vi "7-19-19 increasing temp.vi"() -> ()   [LabVIEW 2016]
uses:
  <userlib>/Levylab/LV to ITX/LVtoITX.lvclass
  <vilib>/Analysis/NI_AALPro.lvlib
panel:
  out "G Vs Time 2":cluster{"Data":dbl[], "Data":dbl[]}(graph)
  in  "Path 2":path=path "G:/My Drive/Data/SA40060.20190715.000000.dat"
  out "dG/dt Vs Temp Normalized vs prev":cluster{"Data":dbl[], "Data":dbl[]}[](graph)
  out "dG/dt Vs Temp Normalized vs 275K":cluster{"Data":dbl[], "Data":dbl[]}[](graph)
  out "dG/dt Vs Temp":cluster{"Data":dbl[], "Data":dbl[]}[](graph)
  out "output cluster":cluster{dbl[], dbl[], dbl[], dbl[]}
  out "G2T Vs Temp":cluster{"Data":dbl[], "Data":dbl[]}[](graph)
  out "Data":dbl[][](array[numeric])
  out "G Vs Time":cluster{"Data":dbl[], "Data":dbl[]}[](graph)
  out "Wavenames":string[](array[string])
  in  "Path":path=path "G:/My Drive/Data/SA40060.20190715.000000.dat"
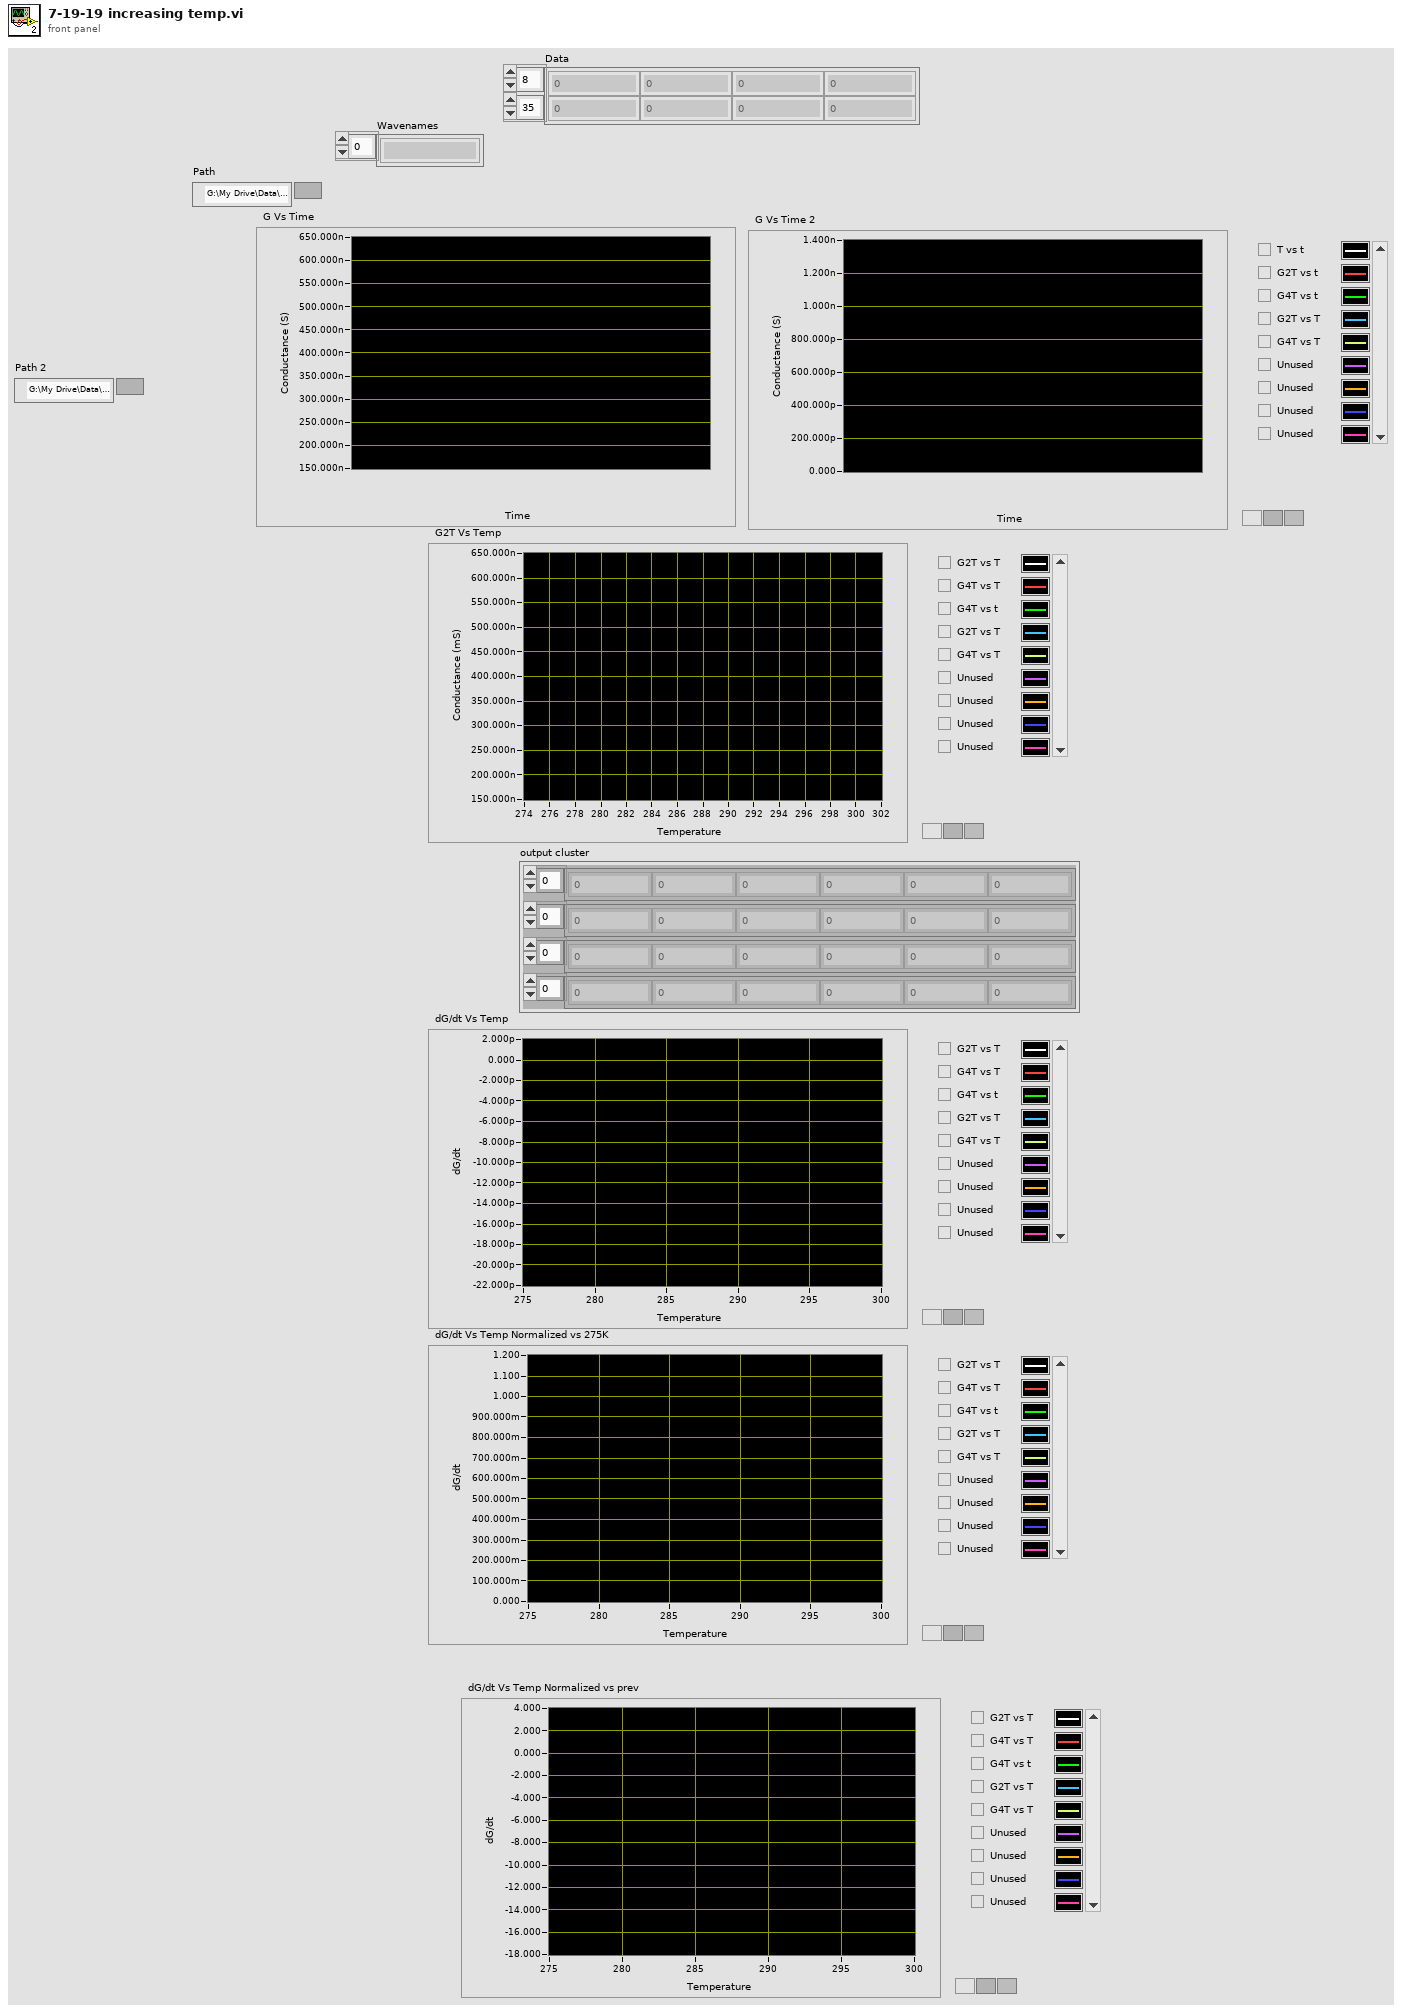
[diagram p1: front panel]
types:
  T1 = cluster{"slope min":dbl, "slope max":dbl, "intercept min":dbl, "intercept max":dbl}
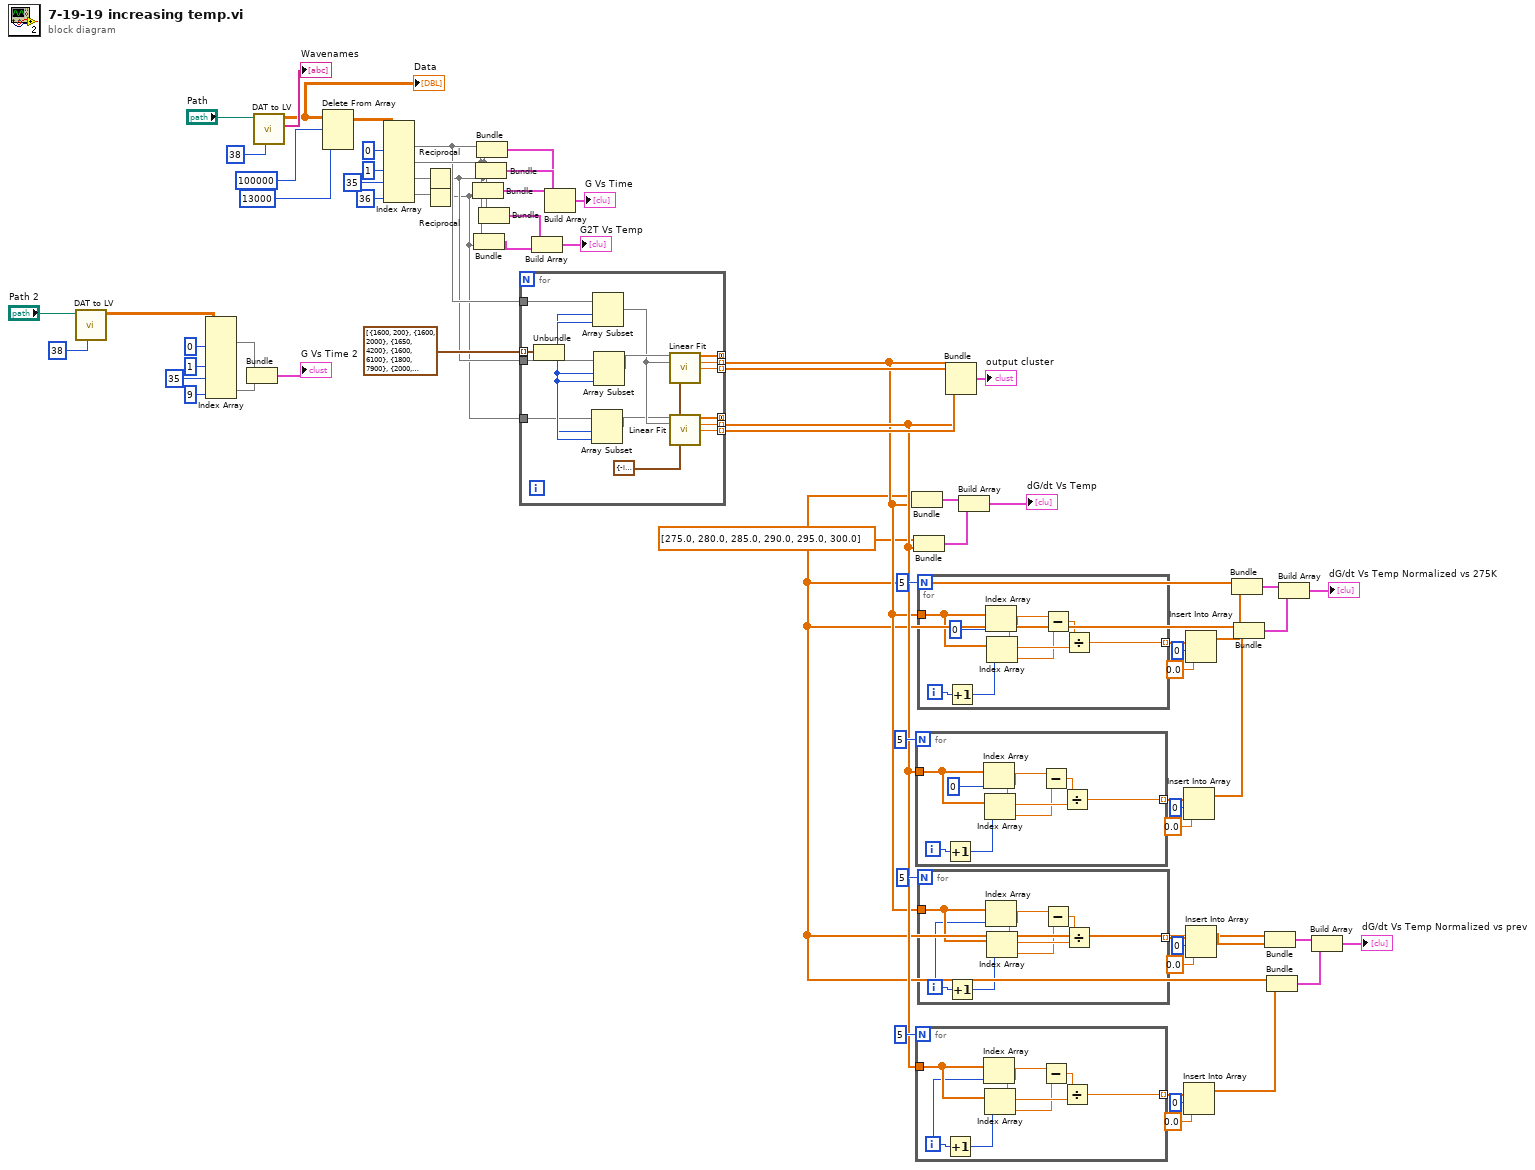
[diagram p0: block diagram]
diagram:
  w11 = dbl[] [275.0, 280.0, 285.0, 290.0, 295.0, 300.0]
  n1 = call <userlib>:"DAT to LV.vi"("header length"=38, "File Path"="Path 2") -> ("Data"=w4:dbl[][])  [unwired: 6 in, 3 out]
  n2 = Index Array(array=w4, index (col) #1=0 ("disabled index (col)"), index (col) #2=1 ("index (col)"), index (col) #3=35 ("index (col)"), index (col) #4=9 ("index (col)")) -> (element #1=w3:dbl[], element #4=w2:dbl[])  [unwired: 4 in, 2 out]
  n3 = Bundle("Data"=w3, "Data"=w2) -> (→"G Vs Time 2":cluster{"Data":dbl[], "Data":dbl[]})  [unwired: 1 in]
  n4 = call <userlib>:"DAT to LV.vi"("header length"=38, "File Path"="Path") -> ("Wavenames"=→"Wavenames":string[], "Data"=w51:dbl[][])  [unwired: 6 in, 2 out]
  "Data" <- w51
  n5 = Delete From Array(array=w51, length=100000, index (row)=13000 ("index")) -> (array with subset deleted=w50:dbl[][])  [unwired: 1 in, 1 out]
  n6 = Index Array(array=w50, index (col) #1=0 ("disabled index (col)"), index (col) #2=1 ("index (col)"), index (col) #3=35 ("index (col)"), index (col) #4=36 ("index (col)")) -> (element #1=w48:dbl[], element #2=w63:dbl[], element #3=w58:dbl[], element #4=w57:dbl[])  [unwired: 4 in]
  n7 = Reciprocal(x=w58) -> (1/x=w47:dbl[])
  n8 = Reciprocal(x=w57) -> (1/x=w46:dbl[])
  n9 = Bundle("Data"=w48, w46) -> (w62:cluster{"Data":dbl[], dbl[]})  [unwired: 1 in]
  n10 = Bundle("Data"=w63, w46) -> (w55:cluster{"Data":dbl[], dbl[]})  [unwired: 1 in]
  n11 = Bundle("Data"=w48, w47) -> (w61:cluster{"Data":dbl[], dbl[]})  [unwired: 1 in]
  n12 = Bundle("Data"=w48, "Data"=w63) -> (w60:cluster{"Data":dbl[], "Data":dbl[]})  [unwired: 1 in]
  n13 = Bundle("Data"=w63, w47) -> (w56:cluster{"Data":dbl[], dbl[]})  [unwired: 1 in]
  n14 = for {
    tunnel: cluster{"length":i32, "index":i32}[] [{"length"=1600, "index"=200}, {"length"=1600, "index"=2000}, {"length"=1650, "index"=4200}, {"length"=1600, "index"=6100}, {"length"=1800, "index"=7900}, {"length"=2000, "index"=10000}] -> [w86] mode=indexing
    tunnel: w48 -> [w83]
    tunnel: w47 -> [w82]
    tunnel: w46 -> [w81]
    tunnel: [w76] -> _ mode=concatenating
    tunnel: [w75] -> _ mode=concatenating
    tunnel: [w74] -> w18 mode=indexing
    tunnel: [w73] -> w45 mode=indexing
    tunnel: [w72] -> w17 mode=indexing
    tunnel: [w71] -> w43 mode=indexing
    w77 = T1 {"slope min"=-inf, "slope max"=inf, "intercept min"=-inf, "intercept max"=inf} ("parameter bounds")
    n15 = Unbundle(w86) -> ("length"=w85:i32, "index"=w84:i32)
    n16 = Array Subset(array=w81, index=w84, length=w85) -> (w78:dbl[])
    n17 = Array Subset(array=w83, index=w84, length=w85) -> (w79:dbl[])
    n18 = Array Subset(array=w82, index=w84, length=w85) -> (w80:dbl[])
    n19 = call <vilib>:"Linear Fit.vi"("Y"=w80, "X"=w79, "parameter bounds"=w77) -> ("Best Linear Fit"=w76:dbl[], "slope"=w72:dbl, "intercept"=w71:dbl)  [unwired: 8 in, 2 out]
    n20 = call <vilib>:"Linear Fit.vi"("Y"=w78, "X"=w79, "parameter bounds"=w77) -> ("Best Linear Fit"=w75:dbl[], "slope"=w74:dbl, "intercept"=w73:dbl)  [unwired: 8 in, 2 out]
  }
  n21 = Build Array(w56, w55) -> (→"G2T Vs Temp":cluster{"Data":dbl[], dbl[]}[])
  n22 = Build Array(w60, w61, w62) -> (→"G Vs Time":cluster{"Data":dbl[], "Data":dbl[]}[])
  n23 = Bundle(w11, w17) -> (w41:cluster{dbl[], dbl[]})  [unwired: 1 in]
  n24 = Bundle(w11, w18) -> (w42:cluster{dbl[], dbl[]})  [unwired: 1 in]
  n25 = for {
    N: 5 -> [_]
    tunnel: w18 -> [w94]
    tunnel: [w87] -> w31 mode=indexing
    i -> [w92]
    n26 = Increment(x=w92) -> (x+1=w91:i32)
    n27 = Index Array(array=w94, index=0) -> (element=w89:dbl)
    n28 = Index Array(array=w94, index=w91) -> (element=w88:dbl)
    n29 = Subtract(x=w89, y=w88) -> (x-y=w90:dbl)
    n30 = Divide(x=w90, y=w89) -> (x/y=w87:dbl)
  }
  n31 = for {
    N: 5 -> [_]
    tunnel: w18 -> [w101]
    tunnel: [w96] -> w25 mode=indexing
    i -> [w95]
    n32 = Increment(x=w95) -> (x+1=w100:i32)
    n33 = Index Array(array=w101, index=w95) -> (element=w98:dbl)
    n34 = Index Array(array=w101, index=w100) -> (element=w97:dbl)
    n35 = Subtract(x=w98, y=w97) -> (x-y=w99:dbl)
    n36 = Divide(x=w99, y=w98) -> (x/y=w96:dbl)
  }
  n37 = for {
    N: 5 -> [_]
    tunnel: w17 -> [w109]
    tunnel: [w102] -> w38 mode=indexing
    i -> [w107]
    n38 = Increment(x=w107) -> (x+1=w106:i32)
    n39 = Index Array(array=w109, index=0) -> (element=w104:dbl)
    n40 = Index Array(array=w109, index=w106) -> (element=w103:dbl)
    n41 = Subtract(x=w104, y=w103) -> (x-y=w105:dbl)
    n42 = Divide(x=w105, y=w104) -> (x/y=w102:dbl)
  }
  n43 = for {
    N: 5 -> [_]
    tunnel: w17 -> [w116]
    tunnel: [w111] -> w20 mode=indexing
    i -> [w110]
    n44 = Increment(x=w110) -> (x+1=w115:i32)
    n45 = Index Array(array=w116, index=w110) -> (element=w113:dbl)
    n46 = Index Array(array=w116, index=w115) -> (element=w112:dbl)
    n47 = Subtract(x=w113, y=w112) -> (x-y=w114:dbl)
    n48 = Divide(x=w114, y=w113) -> (x/y=w111:dbl)
  }
  n49 = Bundle(w17, w43, w18, w45) -> (→"output cluster":cluster{dbl[], dbl[], dbl[], dbl[]})  [unwired: 1 in]
  n50 = Build Array(w41, w42) -> (→"dG/dt Vs Temp":cluster{dbl[], dbl[]}[])
  n51 = Insert Into Array(array=w31, index=0, new element=0.0 ("new element/subarray")) -> (w29:dbl[])
  n52 = Insert Into Array(array=w25, index=0, new element=0.0 ("new element/subarray")) -> (w13:dbl[])
  n53 = Insert Into Array(array=w38, index=0, new element=0.0 ("new element/subarray")) -> (w28:dbl[])
  n54 = Insert Into Array(array=w20, index=0, new element=0.0 ("new element/subarray")) -> (w12:dbl[])
  n55 = Bundle(w11, w28) -> (w35:cluster{dbl[], dbl[]})  [unwired: 1 in]
  n56 = Bundle(w11, w29) -> (w34:cluster{dbl[], dbl[]})  [unwired: 1 in]
  n57 = Bundle(w11, w12) -> (w14:cluster{dbl[], dbl[]})  [unwired: 1 in]
  n58 = Bundle(w11, w13) -> (w15:cluster{dbl[], dbl[]})  [unwired: 1 in]
  n59 = Build Array(w35, w34) -> (→"dG/dt Vs Temp Normalized vs 275K":cluster{dbl[], dbl[]}[])
  n60 = Build Array(w14, w15) -> (→"dG/dt Vs Temp Normalized vs prev":cluster{dbl[], dbl[]}[])
